vi "WSVCAP SHL Host TL SPI Write Cycle.vi"(0 "SPI Data Out":u8[][](array[numeric]) format="%.0x", 5 "Socket Mask":u16=1 format="%02x", 7 "Cycle CMD Lengths (bits)":u8[](array[numeric]), 9 "Cycle CMD Delay (ticks)":u32[](array[numeric]), 11 "error in":errorcluster, 13 "Log (T)":bool=TRUE) -> (15 "error out":errorcluster)   [LabVIEW 2012]
uses:
  Type Defs/WSVCAP SHL Function Enum.ctl
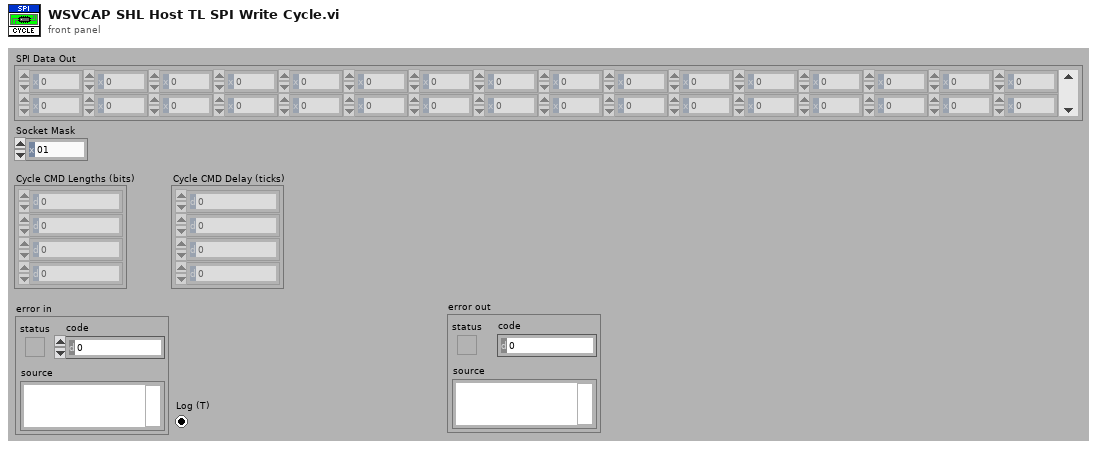
[diagram p1: front panel]
types:
  T1 = typedef "WSVCAP SHL Function Enum.ctl" = enum16{"Initialize", "Configure I2C", "Configure SPI", "Configure RFFE", "Write I2C", "Read I2C", "Write/Read SPI", "Start SPI Cycle", "Stop SPI Cycle", "Write RFFE", "Read RFFE", "Start RFFE Cycle", "Stop RFFE Cycle", "Get Status", "Close"}
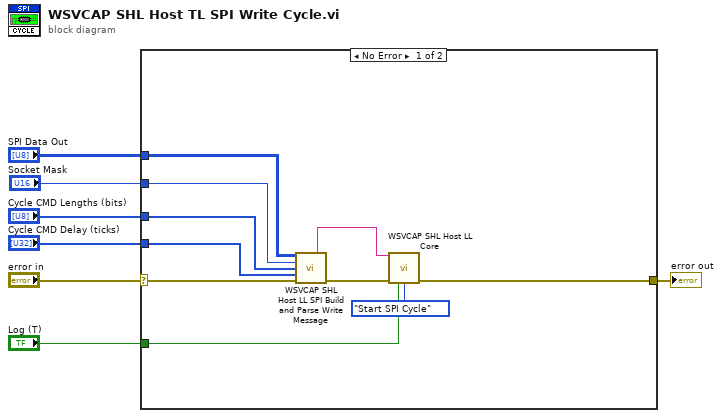
[diagram p0: block diagram]
diagram:
  n1 = case shown="No Error" "error in" {
    selector: "error in" -> [w14 w18]
    tunnel: [w8 w18] -> w7
    tunnel: "SPI Data Out" -> [w13 _]
    tunnel: "Socket Mask" -> [w11 _]
    tunnel: "Log (T)" -> [w12 _]
    tunnel: "Cycle CMD Lengths (bits)" -> [w10 _]
    tunnel: "Cycle CMD Delay (ticks)" -> [w9 _]
    frame No Error {
      n2 = call "WSVCAP SHL Host LL SPI Build and Parse Write Message.vi"("Write Data In [DUT Ordered]"=w13, "Socket Mask [U16] In"=w11, "Cycle CMD Lengths (bits)"=w10, "Cycle CMD Delay (ticks)"=w9, "error in"=w14) -> ("Message Out"=w15:string, "error out"=w16:errorcluster)  [unwired: 5 in, 4 out]
      n3 = call "WSVCAP SHL Host LL Core.vi"("Message In"=w15, "error in"=w16, "Log (T)"=w12, "Function"=WSVCAP_SHL_Function_Enum."Start SPI Cycle") -> ("error out"=w8:errorcluster)  [unwired: 9 in, 2 out]
    }
    frame Error {
    }
  }
  "error out" <- w7
